vi "Build Sample Project - Desktop and RT.vi"(8 "error in (no error)":errorcluster, 11 "Path to project":path=path "C:/Users/design/Documents/LabVIEW Code/ADT Form Processor/ADT Form Processor Project.lvproj") -> (0 "error out":errorcluster, 3 "Generated files":path[][](array[path]))   [LabVIEW 2011, in "Design Server.lvlib"]
uses:
  Design Server.lvlib
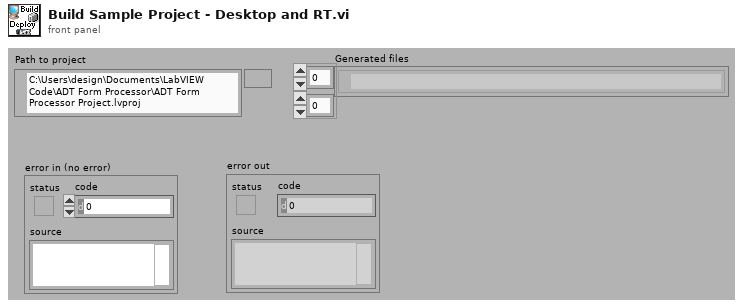
[diagram p1: front panel]
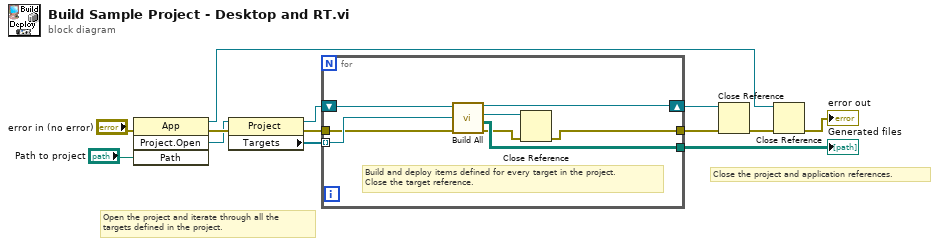
[diagram p0: block diagram]
diagram:
  # "Close the project and application references."
  # "Open the project and iterate through all the\ntargets defined in the project."
  n1 = invoke class="App" method="Project.Open"(error in="error in (no error)", "Path"="Path to project") -> (reference out=w4:refnum<vi>, error out=w12:errorcluster, "Project:Open"=w9:refnum<vi>)  [unwired: 2 in, 1 out]
  n2 = property class="Project"(reference=w9, error in=w12) -> (reference out=w7:refnum<vi>, error out=w10:errorcluster, "Targets"=w11:refnum<vi>[])
  n3 = for {
    tunnel: w11 -> [w20] mode=indexing
    shift-right: [w15] -> w8
    shift-left: w7 -> [w21]
    tunnel: [w17] -> w5
    tunnel: w10 -> [w19]
    tunnel: [w14] -> w2
    # "Build and deploy items defined for every target in the project.\nClose the target reference."
    n4 = call "Build All.vi"("error in"=w19, "TargetItem in"=w20, "Project in"=w21) -> ("error out"=w16:errorcluster, "Generated files"=w17:path[][], "TargetItem out"=w18:refnum<vi>, "Project out"=w15:refnum<vi>)  [unwired: 3 out]
    n5 = Close Reference(reference=w18, error in (no error)=w16) -> (error out=w14:errorcluster)
  }
  "Generated files" <- w5
  n6 = Close Reference(reference=w8, error in (no error)=w2) -> (error out=w13:errorcluster)
  n7 = Close Reference(reference=w4, error in (no error)=w13) -> (error out=→"error out":errorcluster)
